vi "Connect.vi"(8 "error in (no error)":errorcluster, 11 "Connection in":refnum<class "Connection.lvclass">) -> (0 "error out":errorcluster, 3 "Connection out":refnum<class "Connection.lvclass">)   [LabVIEW 2013, in "Connection_GOSPL.lvlib" / "Connection.lvclass"]
uses:
  Connection.lvclass
  connection notifier.ctl
  Connection.lvclass/Connection.ctl
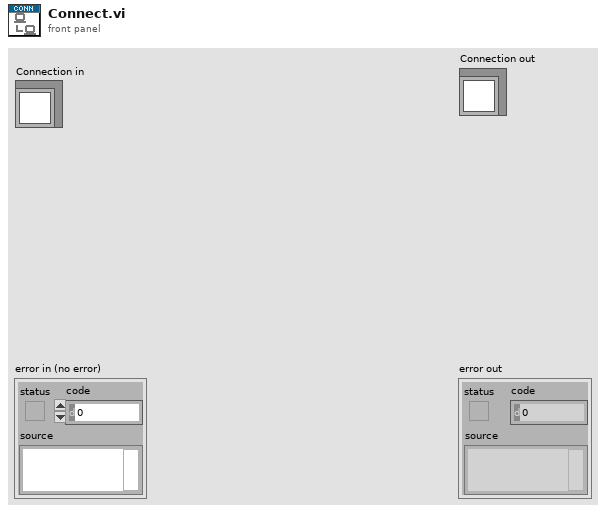
[diagram p1: front panel]
types:
  T1 = typedef "Connection_GOSPL.lvlib/Connection.lvclass/connection notifier.ctl" = cluster{"Connection":refnum<class>, "error":errorcluster}
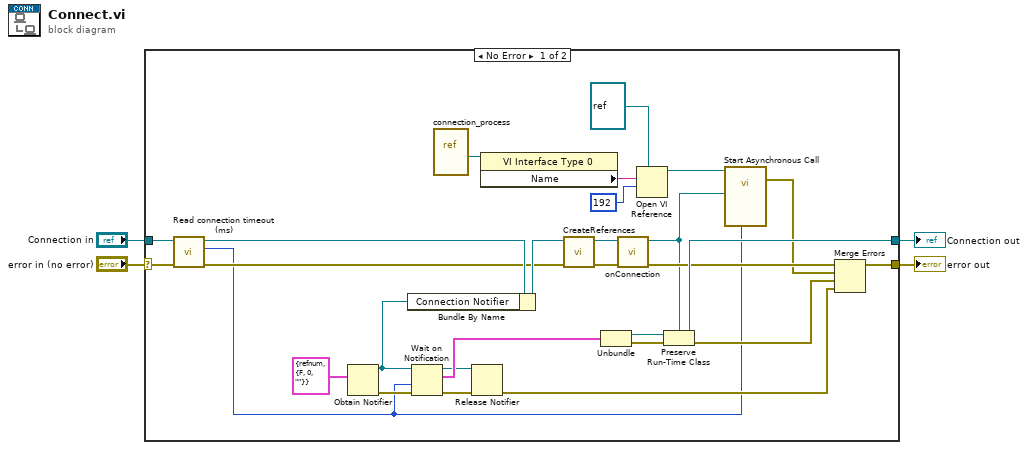
[diagram p0: block diagram]
diagram:
  n1 = case shown="No Error" "error in (no error)" {
    selector: "error in (no error)" -> [w11 w34]
    tunnel: [w30 w34] -> w3
    tunnel: [w17 w33] -> w2
    tunnel: "Connection in" -> [w13 w33]
    frame No Error {
      n2 = call "Read connection timeout (ms).vi"("error in (no error)"=w11, "Connection in"=w13) -> ("error out"=w10:errorcluster, "connection timeout (ms)"=w7:i32, "Connection out"=w12:refnum<class "Connection.lvclass">)  [unwired: 7 in]
      n3 = Obtain Notifier(notification data type=T1 {"Connection"=refnum, "error"={"status"=FALSE, "code"=0, "source"=""}} ("MQTT Server.lvlib:TCPConnection.lvclass:connection notifier")) -> (notifier out=w26:refnum<notifier>, error out=w32:errorcluster)  [unwired: 3 in, 1 out]
      n4 = Bundle By Name(cluster=w12, "Connection Notifier"=w26) -> (w21:refnum<class "Connection.lvclass">)
      n5 = Wait on Notification(notifier=w26, timeout in ms (-1)=w7, error in (no error)=w32) -> (notifier out=w22:refnum<notifier>, notification=w31:T1, error out=w24:errorcluster)  [unwired: 1 in, 1 out]
      n6 = vi-ref "connection_process.vi"() -> (w29:refnum<vi>)
      n7 = Release Notifier(notifier=w22, error in (no error)=w24) -> (error out=w23:errorcluster)  [unwired: 1 in, 2 out]
      n8 = property class="VI Interface Type 0"(reference=w29) -> ("Name"=w28:string)  [unwired: 1 in, 2 out]
      n9 = call-dynamic "CreateReferences.vi"("error in (no error)"=w10, "Connection in"=w21) -> ("error out"=w15:errorcluster, "Connection out"=w16:refnum<class "Connection.lvclass">)  [unwired: 8 in]
      n10 = Unbundle(w31) -> ("Connection"=w20:refnum<class>, "error"=w19:errorcluster)
      n11 = call-dynamic "onConnection.vi"("error in (no error)"=w15, "Connection in"=w16) -> ("error out"=w14:errorcluster, "Connection out"=w8:refnum<class "Connection.lvclass">)  [unwired: 8 in]
      n12 = Open VI Reference(type specifier VI Refnum (for type only)=refnum<vi> refnum, vi path=w28, options=192) -> (vi reference=w5:refnum<vi>)  [unwired: 3 in, 1 out]
      n13 = Preserve Run-Time Class(object in=w20, error in=w19, 2:w8) -> (object out=w17:refnum<class "Connection.lvclass">, error out=w18:errorcluster)
      n14 = call-by-ref "Start Asynchronous Call"(reference=w5, "timeout (ms)"=w7, "Connection"=w8) -> (error out=w6:errorcluster)  [unwired: 11 in, 1 out]
      n15 = Merge Errors(w14, w6, w18, w23) -> (w30:errorcluster)
    }
    frame Error {
    }
  }
  "error out" <- w3
  "Connection out" <- w2
